vi "Append or Replace 1D Array Element (U16).vi"(6 "Default":u16, 8 "Element":u16, 9 "Indices (>=1D)":i32[](array[numeric]), 10 "Index (1D)":i32, 11 "Array In":u16[](array[numeric])) -> (3 "Array Out":u16[](array[numeric]))   [LabVIEW 2009]
doc: "Appends or replaces the array element at given indices. Inefficient for large arrays."
panel:
  # "Append or Replace Array Element.vi\n\nAppends or replaces the array element at given indices.  Inefficient for large arrays.  Currently implemented only for 1D and 2D arrays.\n\nPlease visit http://www.OpenG.org to learn about the\nOpen Source LabVIEW software movement.\n\nNOTICE -- YOU MUST LEAVE THIS NOTICE IN PLACE.  PER THE TERMS OF THE LICENSE BELOW, YOU MAY SUBLICENSE THIS SOFTWARE \nIN ANY WAY THAT DOES NOT CONFLICT WITH THIS LICENSE.\n\n### BSD License (http://www.opensource.org/licenses/bsd-license.php) Begin ###\n \nCopyright (c) 2005, MKS Instruments, Inc., author: Doug Femec<doug_femec@mksinst.com>, IM dafemec\n\nAll rights reserved.\n\nRedistribution and use in source and binary forms, with or without modification, are permitted provided that the following conditions are met:\n\n    * Redistributions of source code must retain the above copyright notice, this list of conditions and the following disclaimer.\n    * Redistributions in binary form must reproduce the above copyright notice, this list of conditions and the following disclaimer in the \n       documentation and/or other materials provided with the distribution.\n    * Neither the name of SciWare, James Kring, Inc., nor the names of its contributors may be used to endorse or promote products derived \n       from this software without specific prior written permission.\n\nTHIS SOFTWARE IS PROVIDED BY THE COPYRIGHT HOLDERS AND CONTRIBUTORS \"AS IS\" AND ANY EXPRESS OR IMPLIED WARRANTIES, \nINCLUDING, BUT NOT LIMITED TO, THE IMPLIED WARRANTIES OF MERCHANTABILITY AND FITNESS FOR A PARTICULAR PURPOSE ARE \nDISCLAIMED. IN NO EVENT SHALL THE COPYRIGHT OWNER OR CONTRIBUTORS BE LIABLE FOR ANY DIRECT, INDIRECT, INCIDENTAL,\n SPECIAL, EXEMPLARY, OR CONSEQUENTIAL DAMAGES (INCLUDING, BUT NOT LIMITED TO, PROCUREMENT OF SUBSTITUTE GOODS OR \nSERVICES; LOSS OF USE, DATA, OR PROFITS; OR BUSINESS INTERRUPTION) HOWEVER CAUSED AND ON ANY THEORY OF LIABILITY, \nWHETHER IN CONTRACT, STRICT LIABILITY, OR TORT (INCLUDING NEGLIGENCE OR OTHERWISE) ARISING IN ANY WAY OUT OF THE USE \nOF THIS SOFTWARE, EVEN IF ADVISED OF THE POSSIBILITY OF SUCH DAMAGE.\n\n### BSD License End ###"
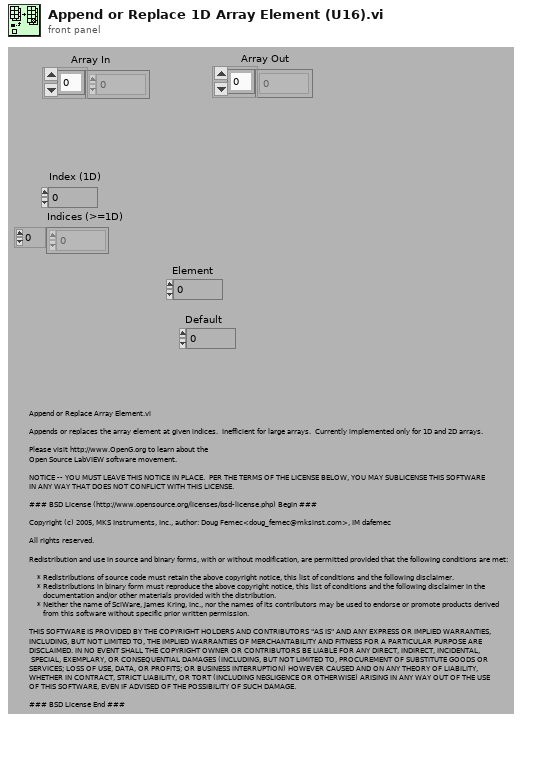
[diagram p1: front panel]
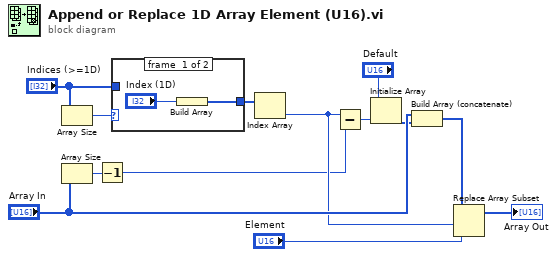
[diagram p0: block diagram]
diagram:
  n1 = Array Size(array="Indices (>=1D)") -> (size(s)=w11:i32)
  n2 = Array Size(array="Array In") -> (size(s)=w8:i32)
  n3 = Decrement(x=w8) -> (x-1=w2:i32)
  n4 = case shown="0" w11 {
    tunnel: [w14 w16] -> w9
    tunnel: "Indices (>=1D)" -> [_ w16]
    frame #0 {
      n5 = Build Array("Index (1D)") -> (w14:i32[])
    }
    frame #1 {
    }
  }
  n6 = Index Array(array=w9) -> (element=w3:i32)  [unwired: 1 in]
  n7 = Subtract(x=w3, y=w2) -> (x-y=w7:i32)
  n8 = Initialize Array("Default", w7) -> (w6:u16[])
  n9 = Build Array (concatenate)("Array In", w6) -> (w1:u16[])
  n10 = Replace Array Subset(array=w1, new element="Element", index=w3) -> (→"Array Out":u16[])
